vi "test Initialize Engine Pointer.vi"(8 "error in (no error)":errorcluster, 11 "TestCase in":refnum<class "Framework Property Tests.lvclass">) -> (0 "error out":errorcluster, 3 "TestCase out":refnum<class "Framework Property Tests.lvclass">)   [LabVIEW 2017, in "Framework Property Tests.lvclass"]
uses:
  Framework Property Tests.lvclass
  <vilib>/addons/_JKI Toolkits/VI Tester/TestCase.llb/TestCase.lvclass
  Classes/Framework/Framework.lvclass
  LabVIEW-Memory/Source/Classes/Pointer/Pointer.lvclass
  LabVIEW-Memory/Source/Classes/Pointer/Write Bool.vi
  LabVIEW-Memory/Source/Classes/Pointer/Read Bool.vi
  C:/Program Files (x86)/National Instruments/LabVIEW 2017/vi.lib/addons/_JKI Toolkits/VI Tester/TestCase.llb/TestCase.lvclass
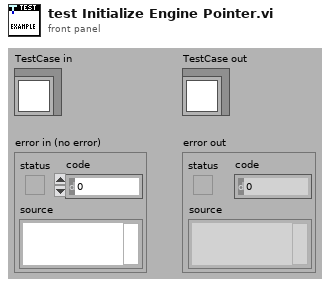
[diagram p1: front panel]
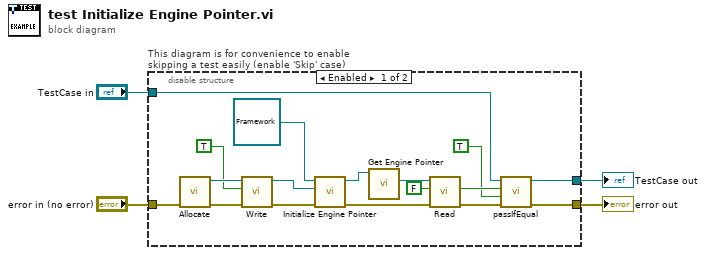
[diagram p0: block diagram]
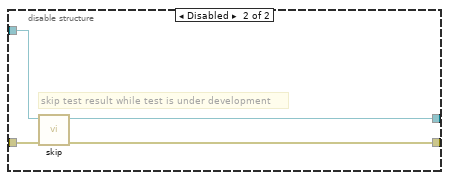
[diagram p2: hidden frame]
diagram:
  n1 = disable-structure "This diagram is for convenience to enable skipping a test easily (enable 'Skip' case)" shown="Enabled" {
    disable-tunnel: "TestCase in" -> [w8 w25]
    disable-tunnel: [w7 w23] -> w1
    disable-tunnel: [w9 w24] -> w3
    disable-tunnel: "error in (no error)" -> [w14 w22]
    frame Enabled {
      n2 = call "Allocate.vi"("error in (no error)"=w14) -> ("error out"=w13:errorcluster, "Pointer out"=w20:refnum<class "Pointer.lvclass">)  [unwired: 9 in]
      n3 = call-poly "Write.vi"("error in (no error)"=w13, "value"=TRUE, "Pointer in"=w20) -> ("error out"=w12:errorcluster, "Pointer out"=w19:refnum<class "Pointer.lvclass">)  [unwired: 5 in, 2 out]
      n4 = call "Initialize Engine Pointer.vi"("error in (no error)"=w12, "Engine Pointer"=w19, "Framework in"=refnum<class "Framework.lvclass"> refnum) -> ("error out"=w11:errorcluster, "Framework out"=w17:refnum<class "Framework.lvclass">)  [unwired: 7 in]
      n5 = call "Get Engine Pointer.vi"("Framework in"=w17) -> ("Engine Pointer"=w16:refnum<class "Pointer.lvclass">)  [unwired: 9 in, 1 out]
      n6 = call-poly "Read.vi"("error in (no error)"=w11, "value in"=FALSE, "Pointer in"=w16) -> ("error out"=w10:errorcluster, "value out"=w6:bool)  [unwired: 5 in, 2 out]
      n7 = call-dynamic "passIfEqual.vi"("error in (no error)"=w10, "y"=TRUE ("value out"), "x"=w6, "TestCase in"=w8) -> ("error out"=w9:errorcluster, "TestCase out"=w7:refnum<class "Framework Property Tests.lvclass">)  [unwired: 6 in]
    }
    frame Disabled {
      # "skip test result while test is under development"
      n8 = call <vilib>:"skip.vi"("error in (no error)"=w22, "TestCase in"=w25) -> ("error out"=w24:errorcluster, "TestCase out"=w23:refnum<class "Framework Property Tests.lvclass">)  [unwired: 8 in]
    }
  }
  "error out" <- w3
  "TestCase out" <- w1
